vi "RageATE_Send Email Attachment_2.vi"(0 "To: (email@site.com)":string[](array[string]), 1 "Subject:":string="LV SMTP", 3 "Body:":string="testing empty attachment path", 4 "Attachment Path":path[](array[path]), 5 "error in (no error)":errorcluster, 6 "SMTP Outgoing Mail Server":string="smtp.office365.com", 7 "Port":i32=587, 9 "Send Attachment(t)":bool, 10 "From: (email@site.com)":string="tomw@ragesystems.com", 11 "Email Account ID":string="tomw@ragesystems.com", 13 "Email Account Password":string="175CabotSt!") -> (19 "error out":errorcluster)   [LabVIEW 2018]
uses:
  <vilib>/smtpClient/Set Message Text Html.vi
  <vilib>/smtpClient/LabVIEWSMTPClient.lvlib
panel:
  # "Overview: This example shows how to send email attachments from LabVIEW using any SMTP email service, such as Gmail.\nRequirements: LabVIEW 2012 (or compatible)\nInstructions: \n1. Configure all the controls on the front panel. If you use a Gmail account, set SMTP Outgping Mail Server to smtp.gmail.com\n2. Run the VI"
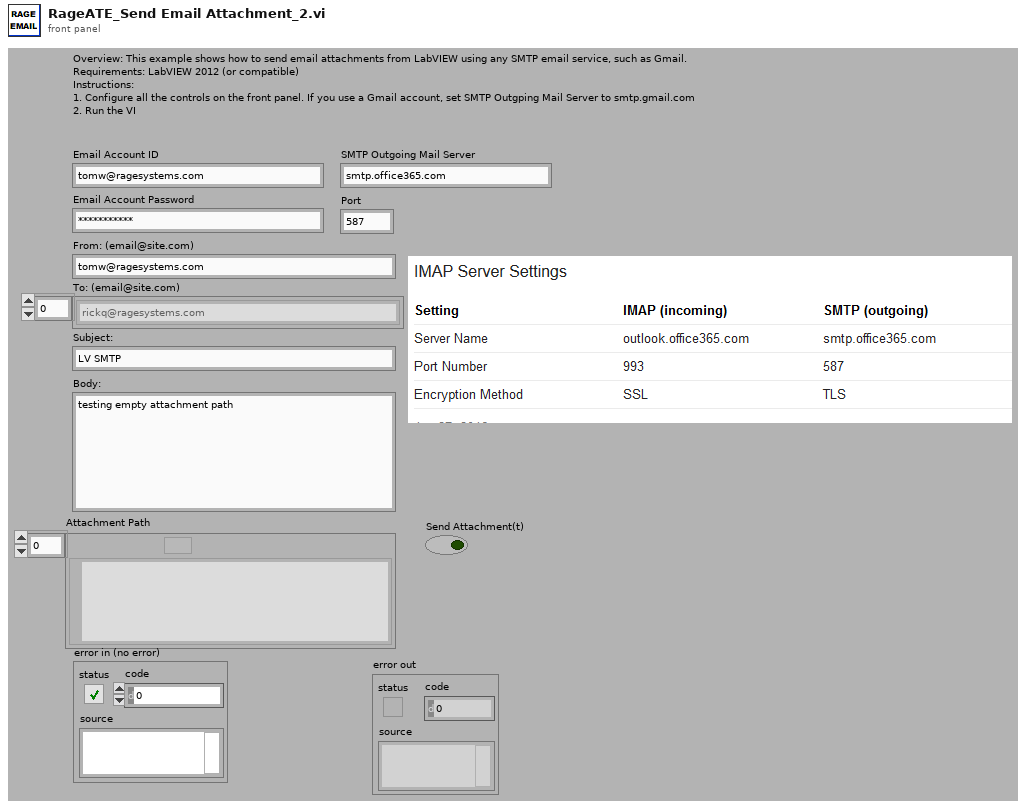
[diagram p1: front panel]
types:
  T1 = typedef "LabVIEWSMTPClient.lvlib/SmtpClientHandle.ctl" = refnum<k1>
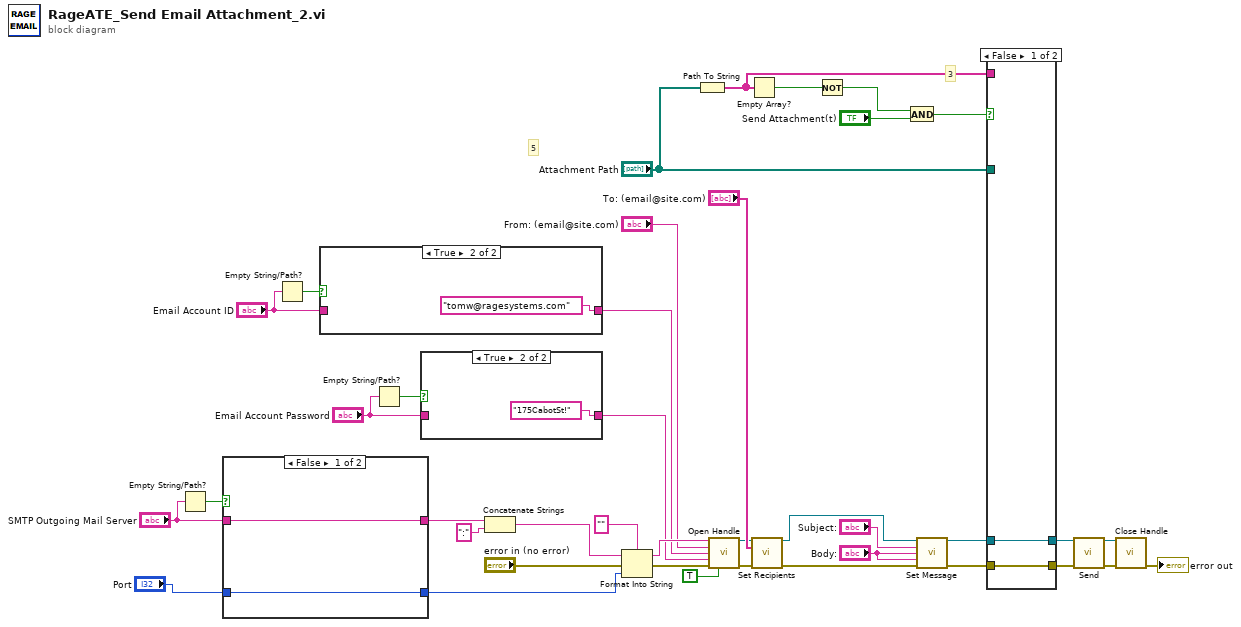
[diagram p0: block diagram]
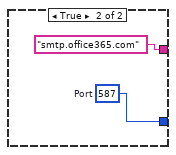
[diagram p2: hidden frame]
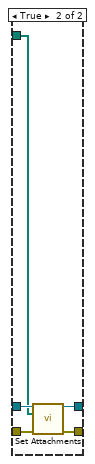
[diagram p5: hidden frame]
diagram:
  # "5"
  # "3"
  n1 = Empty String/Path?(string/path="SMTP Outgoing Mail Server") -> (empty?=w5:bool)
  n2 = case shown="False" w5 {
    tunnel: [w41 "smtp.office365.com" ("SMTP Outgoing Mail Server")] -> w4
    tunnel: "SMTP Outgoing Mail Server" -> [w41 _]
    tunnel: [w40 w42] -> w2
    tunnel: "Port" -> [w40 _]
    frame False {
    }
    frame True {
      w42 = 587  # Port
    }
  }
  n3 = Empty String/Path?(string/path="Email Account ID") -> (empty?=w9:bool)
  n4 = case shown="True" w9 {
    tunnel: [w44 "tomw@ragesystems.com" ("Email Account ID")] -> w11
    tunnel: "Email Account ID" -> [w44 _]
    frame False {
    }
    frame True {
    }
  }
  n5 = Empty String/Path?(string/path="Email Account Password") -> (empty?=w7:bool)
  n6 = case shown="True" w7 {
    tunnel: [w46 "175CabotSt!" ("Email Account Password 2")] -> w8
    tunnel: "Email Account Password" -> [w46 _]
    frame False {
    }
    frame True {
    }
  }
  n7 = Concatenate Strings(w4, ":" ("string")) -> (w37:string)
  n8 = Format Into String(format string="", initial string=w37, error in="error in (no error)", w2) -> (resulting string=w35:string, error out=w17:errorcluster)
  n9 = Path To String(path="Attachment Path") -> (string=w39:string[])
  n10 = call <vilib>:"Open Handle.vi"("server address"=w35, "from"="From: (email@site.com)", "username"=w11, "password"=w8, "error in (no error)"=w17, "use TLS (false)"=TRUE) -> ("handle out"=w31:T1, "error out"=w26:errorcluster)  [unwired: 8 in]
  n11 = Empty Array?(array=w39) -> (empty?=w27:bool)
  n12 = call <vilib>:"Set Recipients.vi"("handle in"=w31, "to"="To: (email@site.com)", "error in (no error)"=w26) -> ("handle out"=w30:T1, "error out"=w25:errorcluster)  [unwired: 11 in]
  n13 = Not(x=w27) -> (.not. x?=w15:bool)
  n14 = And(x=w15, y="Send Attachment(t)") -> (x .and. y?=w14:bool)
  n15 = call-poly <vilib>:"Set Message.vi"("handle in"=w30, "subject"="Subject:", "plain text message"="Body:", "html message"="Body:", "error in (no error)"=w25) -> ("handle out"=w29:T1, "error out"=w24:errorcluster)  [unwired: 9 in]
  n16 = case shown="False" w14 {
    tunnel: w29 -> [w49 w54]
    tunnel: w39 -> [_ _]
    tunnel: "Attachment Path" -> [_ w53]
    tunnel: w24 -> [w48 w52]
    tunnel: [w49 w51] -> w23
    tunnel: [w48 w50] -> w22
    frame False {
    }
    frame True {
      n17 = call <vilib>:"Set Attachments.vi"("handle in"=w54, "attachments"=w53, "error in (no error)"=w52) -> ("handle out"=w51:T1, "error out"=w50:errorcluster)  [unwired: 11 in]
    }
  }
  n18 = call <vilib>:"Send.vi"("handle in"=w23, "error in (no error)"=w22) -> ("handle out"=w20:T1, "error out"=w21:errorcluster)  [unwired: 11 in, 1 out]
  n19 = call <vilib>:"Close Handle.vi"("handle in"=w20, "error in (no error)"=w21) -> ("error out"=→"error out":errorcluster)  [unwired: 12 in, 1 out]
